vi "Decode Date-Time Tag (Erroneous Type).vi"(8 "error in (no error)":errorcluster, 11 "PicoQuant Tag":T1 {"TagType" format="%.0x"}) -> (0 "error out":errorcluster, 3 "Creation Time":string)   [LabVIEW 2021, in "PTU Files.lvlib"]
uses:
  PTU Files.lvlib
  PicoQuant Header Tag.ctl
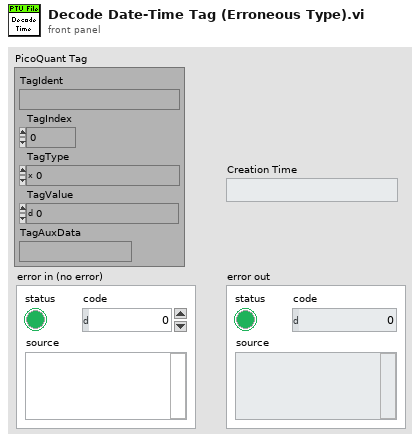
[diagram p1: front panel]
types:
  T1 = typedef "PTU Files.lvlib/PicoQuant Header Tag.ctl" = cluster{"TagIdent":string, "TagIndex":i32, "TagType":i32, "TagValue":i64, "TagAuxData":string}
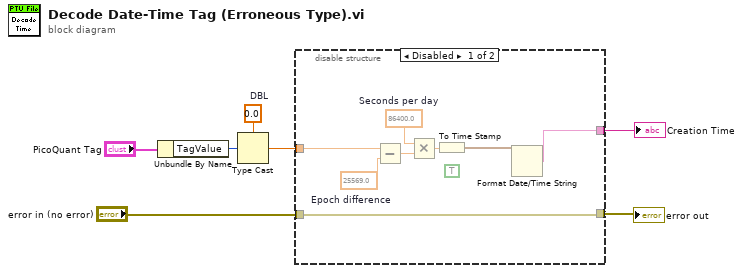
[diagram p0: block diagram]
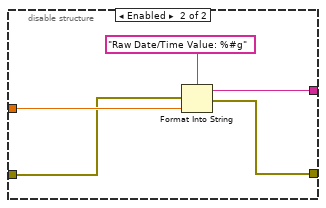
[diagram p2: hidden frame]
diagram:
  w6 = 0.0  # DBL
  n1 = Unbundle By Name("PicoQuant Tag") -> ("TagValue"=w3:i64)
  n2 = Type Cast(type=w6, x=w3) -> (*(type *) &x=w5:dbl)
  n3 = disable-structure shown="Disabled" {
    disable-tunnel: w5 -> [w10 w19]
    disable-tunnel: [w9 w16] -> w4
    disable-tunnel: "error in (no error)" -> [w8 w18]
    disable-tunnel: [w8 w17] -> w1
    frame Disabled {
      (unwired) TRUE ("UTC format")
      w13 = 86400.0  # Seconds per day
      w15 = 25569.0  # Epoch difference
      n4 = Subtract(x=w10, y=w15) -> (x-y=w14:dbl)
      n5 = Multiply(x=w13, y=w14) -> (x*y=w12:dbl)
      n6 = To Time Stamp(1:w12) -> (0:w11:timestamp)
      n7 = Format Date/Time String(seconds (now)=w11) -> (date/time string=w9:string)  [unwired: 2 in]
    }
    frame Enabled {
      n8 = Format Into String(format string="Raw Date/Time Value: %#g" ("date/time string"), error in=w18, w19) -> (resulting string=w16:string, error out=w17:errorcluster)  [unwired: 1 in]
    }
  }
  "Creation Time" <- w4
  "error out" <- w1
